vi "WPI_Robot6DriveMotors.vi"(8 "error in (no error)":errorcluster, 9 "RightSpeed":dbl, 10 "LeftSpeed":dbl, 11 "RobotDriveDevRef":T1={"DevStatus"={"status"=FALSE, "code"=0, "source"=""}, "Motors[]"=[], "Square Inputs"=FALSE, "Max Output"=1.0, "Isochronous"=FALSE}) -> (0 "error out":errorcluster, 2 "Motor Values":dbl[](array[numeric]), 3 "RobotDriveDevRef":T1={"DevStatus"={"status"=FALSE, "code"=0, "source"=""}, "Motors[]"=[], "Square Inputs"=FALSE, "Max Output"=1.0, "Isochronous"=FALSE})   [LabVIEW 2013]
doc: "Determines the motor configuration and sends the speed values to the appropriate motors.\n\nThis software is licensed. Open the labview\\readme\\WPI Robotics Library Open Source License.txt file for more information."
uses:
  <vilib>/Rock Robotics/WPI/RobotDrive/WPI_RobotDriveDevRef.ctl
  <vilib>/Rock Robotics/WPI/MotorControl/WPI_MotorControlDeviceRef.ctl
  <vilib>/Rock Robotics/SystemInterfaces/Typedef/FPGA_TypedefDigitalModule.ctl
  <vilib>/Rock Robotics/SystemInterfaces/DIO/FPGA_DIOPWMChannel.ctl
  <vilib>/Rock Robotics/WPI/PWM/WPI_PWMDeadband.ctl
  <vilib>/Rock Robotics/WPI/CAN/Jaguar/SubVIs/WPI_CANJaguar_ControlMode.ctl
  <vilib>/Rock Robotics/WPI/PWM/WPI_PWMTransform_ConPane.ctl
  WPI_RobotDriveMotorSelectorEnum.ctl
  <vilib>/Rock Robotics/WPI/RobotDrive/WPI_RobotDriveSafetyCheck.vi
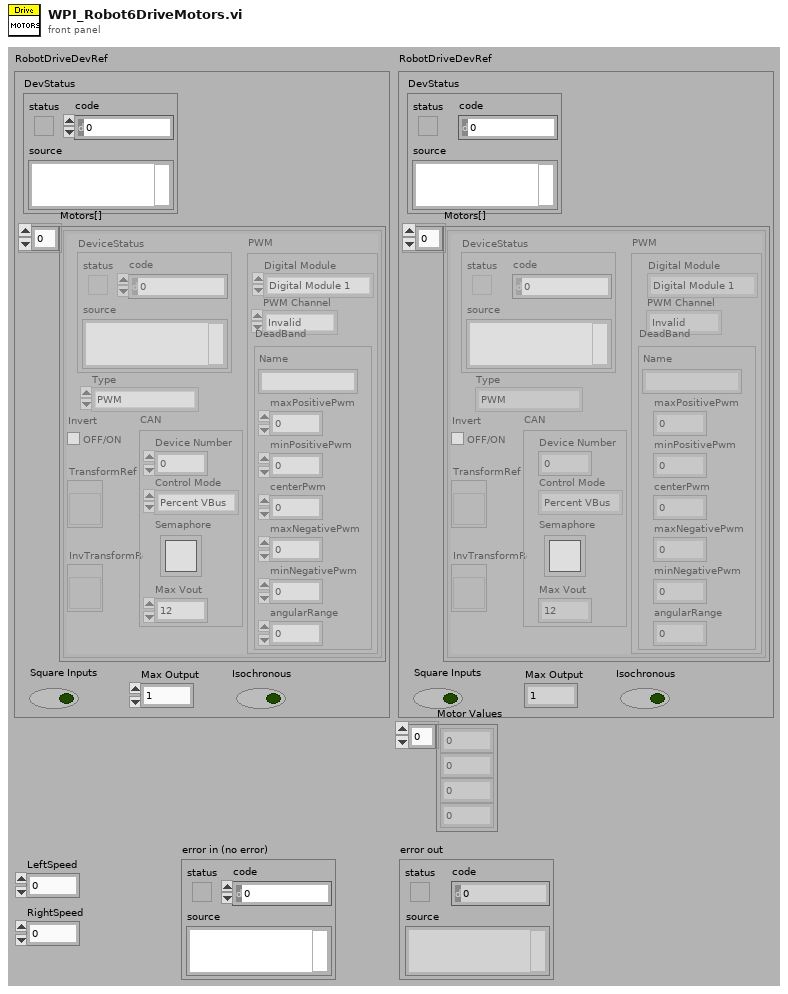
[diagram p1: front panel]
types:
  T1 = typedef "WPI_RobotDriveDevRef.ctl" = cluster{"DevStatus":errorcluster, "Motors[]":T2[], "Square Inputs":bool, "Max Output":dbl, "Isochronous":bool}
  T2 = typedef "WPI_MotorControlDeviceRef.ctl" = cluster{"DeviceStatus":errorcluster, "Type":enum16{"PWM", "CAN"}, "PWM":cluster{"Digital Module":T3, "PWM Channel":T4, "DeadBand":T5}, "CAN":cluster{"Device Number":u8, "Control Mode":T6, "Semaphore":T7, "Max Vout":dbl}, "Invert":bool, "TransformRef":T8, "InvTransformRef":T8}
  T3 = typedef "FPGA_TypedefDigitalModule.ctl" = enum16{"Digital Module 1", "Digital Module 2"}
  T4 = typedef "FPGA_DIOPWMChannel.ctl" = enum8{"PWM 1", "PWM 2", "PWM 3", "PWM 4", "PWM 5", "PWM 6", "PWM 7", "PWM 8", "PWM 9", "PWM 10", "Invalid"}
  T5 = typedef "WPI_PWMDeadband.ctl" = cluster{"Name":string, "maxPositivePwm":i32, "minPositivePwm":i32, "centerPwm":i32, "maxNegativePwm":i32, "minNegativePwm":i32, "angularRange":u16}
  T6 = typedef "WPI_CANJaguar_ControlMode.ctl" = enum8{"Percent VBus", "Current", "Speed", "Position", "Voltage"}
  T7 = typedef "Semaphore RefNum" = refnum<k1>
  T8 = typedef "WPI_PWMTransform_ConPane.ctl" = refnum<vi>
  T9 = typedef "WPI_RobotDriveMotorSelectorEnum.ctl" = enum16{"Rear Left Motor", "Rear Right Motor", "Front Left Motor", "Front Right Motor", "Mid Left Motor", "Mid Right Motor", ""}
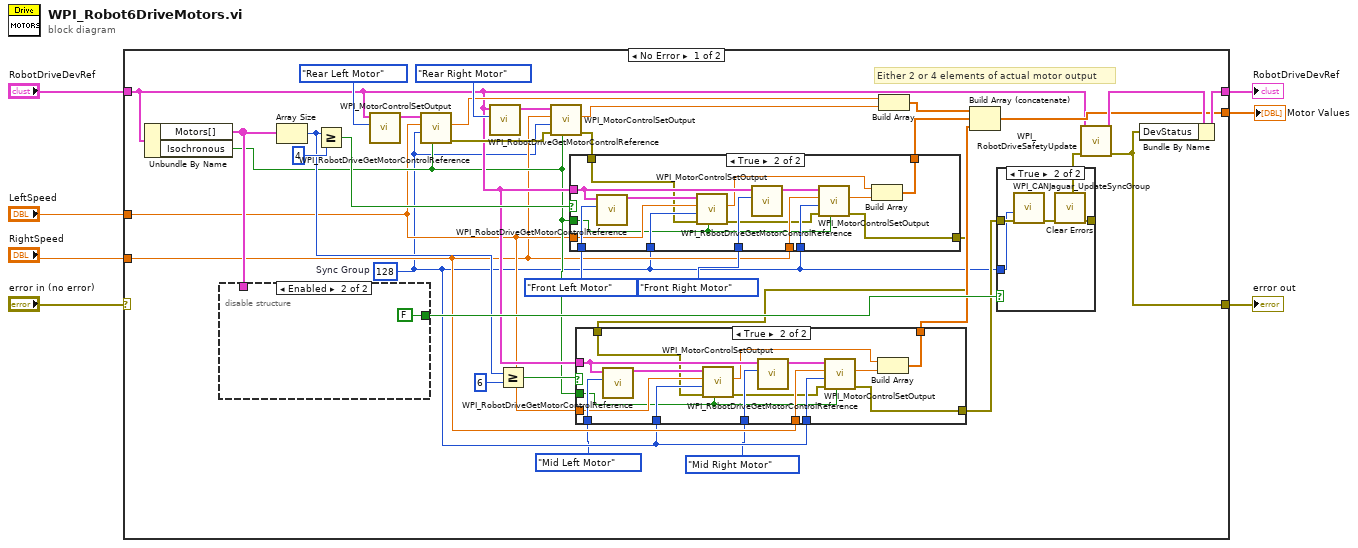
[diagram p0: block diagram]
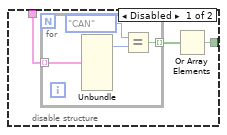
[diagram p2: hidden frame]
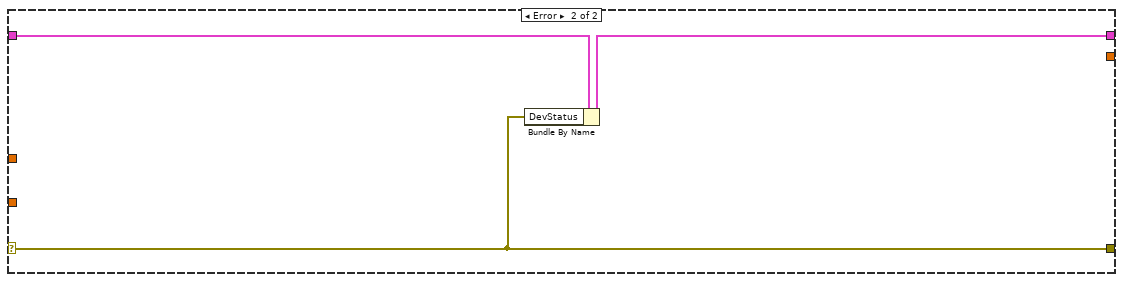
[diagram p6: hidden frame]
diagram:
  n1 = case shown="No Error" "error in (no error)" {
    selector: "error in (no error)" -> [_ w90]
    tunnel: "RobotDriveDevRef" -> [w18 w91]
    tunnel: [w32 w89] -> w6
    tunnel: "LeftSpeed" -> [w13 _]
    tunnel: "RightSpeed" -> [w12 _]
    tunnel: [w33 w90] -> w2
    tunnel: [w21 _] -> w1
    frame No Error {
      w11 = u8 128  # Sync Group
      # "Either 2 or 4 elements of actual motor output"
      n2 = Unbundle By Name(w18) -> ("Motors[]"=w30:T2[], "Isochronous"=w14:bool)
      n3 = disable-structure shown="Enabled" {
        disable-tunnel: w30 -> [w44 _]
        disable-tunnel: [w42 FALSE] -> w29
        frame Disabled {
          n4 = for {
            tunnel: w44 -> [w48] mode=indexing
            tunnel: [w45] -> w43 mode=indexing
            n5 = Unbundle(w48) -> ("Type"=w47:enum16{"PWM", "CAN"})  [unwired: 6 out]
            n6 = Equal?(x=enum16{"PWM", "CAN"}."CAN" ("Type"), y=w47) -> (x = y?=w45:bool)
          }
          n7 = Or Array Elements(Boolean array=w43) -> (logical OR=w42:bool)
        }
        frame Enabled {
        }
      }
      n8 = Array Size(array=w30) -> (size(s)=w19:i32)
      n9 = Greater Or Equal?(x=w19, y=4) -> (x >= y?=w31:bool)
      n10 = call <vilib>:"WPI_RobotDriveGetMotorControlReference.vi"("MotorIndex"=WPI_RobotDriveMotorSelectorEnum."Rear Left Motor", "RobotDriveDevRef"=w18) -> ("MotorControlDeviceRef"=w39:T2)  [unwired: 9 out]
      n11 = call <vilib>:"WPI_MotorControlSetOutput.vi"("Isochronous"=w14, "Sync Group"=w11, "Output"=w13, "MotorControlDevRef"=w39) -> ("error out"=w28:errorcluster, "Motor Output"=w25:dbl)  [unwired: 1 in, 5 out]
      n12 = call <vilib>:"WPI_RobotDriveGetMotorControlReference.vi"("MotorIndex"=WPI_RobotDriveMotorSelectorEnum."Rear Right Motor", "RobotDriveDevRef"=w18) -> ("MotorControlDeviceRef"=w40:T2)  [unwired: 9 out]
      n13 = Greater Or Equal?(x=w19, y=6) -> (x >= y?=w20:bool)
      n14 = call <vilib>:"WPI_MotorControlSetOutput.vi"("Isochronous"=w14, "error in (no error)"=w28, "Sync Group"=w11, "Output"=w12, "MotorControlDevRef"=w40) -> ("error out"=w27:errorcluster, "Motor Output"=w24:dbl)  [unwired: 5 out]
      n15 = case shown="True" w31 {
        tunnel: WPI_RobotDriveMotorSelectorEnum."Front Left Motor" ("MotorIndex") -> [_ w88]
        tunnel: WPI_RobotDriveMotorSelectorEnum."Front Right Motor" ("MotorIndex") -> [_ w87]
        tunnel: w18 -> [_ w86]
        tunnel: w11 -> [_ w85]
        tunnel: w12 -> [_ w84]
        tunnel: w13 -> [_ w83]
        tunnel: [w72 w78] -> w16
        tunnel: w11 -> [_ w80]
        tunnel: w14 -> [_ w79]
        tunnel: w27 -> [w72 w76]
        tunnel: [_ w73] -> w23
        frame False {
        }
        frame True {
          n16 = call <vilib>:"WPI_RobotDriveGetMotorControlReference.vi"("MotorIndex"=w88, "RobotDriveDevRef"=w86) -> ("MotorControlDeviceRef"=w81:T2)  [unwired: 9 out]
          n17 = call <vilib>:"WPI_MotorControlSetOutput.vi"("Isochronous"=w79, "error in (no error)"=w76, "Sync Group"=w80, "Output"=w83, "MotorControlDevRef"=w81) -> ("error out"=w77:errorcluster, "Motor Output"=w74:dbl)  [unwired: 5 out]
          n18 = call <vilib>:"WPI_RobotDriveGetMotorControlReference.vi"("MotorIndex"=w87, "RobotDriveDevRef"=w86) -> ("MotorControlDeviceRef"=w82:T2)  [unwired: 9 out]
          n19 = call <vilib>:"WPI_MotorControlSetOutput.vi"("Isochronous"=w79, "error in (no error)"=w77, "Sync Group"=w85, "Output"=w84, "MotorControlDevRef"=w82) -> ("error out"=w78:errorcluster, "Motor Output"=w75:dbl)  [unwired: 5 out]
          n20 = Build Array(w74, w75) -> (w73:dbl[])
        }
      }
      n21 = case shown="True" w20 {
        tunnel: WPI_RobotDriveMotorSelectorEnum."Mid Left Motor" ("MotorIndex") -> [_ w66]
        tunnel: WPI_RobotDriveMotorSelectorEnum."Mid Right Motor" ("MotorIndex") -> [_ w65]
        tunnel: w18 -> [_ w64]
        tunnel: w11 -> [_ w63]
        tunnel: w12 -> [_ w62]
        tunnel: w13 -> [_ w61]
        tunnel: [w50 w56] -> w15
        tunnel: w11 -> [_ w58]
        tunnel: w14 -> [_ w57]
        tunnel: w16 -> [w50 w54]
        tunnel: [_ w51] -> w17
        frame False {
        }
        frame True {
          n22 = call <vilib>:"WPI_RobotDriveGetMotorControlReference.vi"("MotorIndex"=w66, "RobotDriveDevRef"=w64) -> ("MotorControlDeviceRef"=w59:T2)  [unwired: 9 out]
          n23 = call <vilib>:"WPI_MotorControlSetOutput.vi"("Isochronous"=w57, "error in (no error)"=w54, "Sync Group"=w58, "Output"=w61, "MotorControlDevRef"=w59) -> ("error out"=w55:errorcluster, "Motor Output"=w52:dbl)  [unwired: 5 out]
          n24 = call <vilib>:"WPI_RobotDriveGetMotorControlReference.vi"("MotorIndex"=w65, "RobotDriveDevRef"=w64) -> ("MotorControlDeviceRef"=w60:T2)  [unwired: 9 out]
          n25 = call <vilib>:"WPI_MotorControlSetOutput.vi"("Isochronous"=w57, "error in (no error)"=w55, "Sync Group"=w63, "Output"=w62, "MotorControlDevRef"=w60) -> ("error out"=w56:errorcluster, "Motor Output"=w53:dbl)  [unwired: 5 out]
          n26 = Build Array(w52, w53) -> (w51:dbl[])
        }
      }
      n27 = Build Array(w25, w24) -> (w22:dbl[])
      n28 = Build Array (concatenate)(w22, w23, w17) -> (w21:dbl[])
      n29 = case shown="True" w29 {
        tunnel: w15 -> [w67 w70]
        tunnel: w11 -> [_ w69]
        tunnel: [w67 w68] -> w26
        frame False {
        }
        frame True {
          n30 = call <vilib>:"WPI_CANJaguar_UpdateSyncGroup.vi"("error in (no error)"=w70, "Sync Group"=w69) -> ("error out"=w71:errorcluster)  [unwired: 9 out]
          n31 = call <vilib>:"Clear Errors.vi"("error in (no error)"=w71) -> ("error out"=w68:errorcluster)  [unwired: 6 out]
        }
      }
      n32 = call <vilib>:"WPI_RobotDriveSafetyUpdate.vi"("error in (no error)"=w26, "RobotDriveDevRef"=w18) -> ("error out"=w33:errorcluster, "RobotDriveDevRef"=w34:T1)  [unwired: 8 out]
      n33 = Bundle By Name(cluster=w34, "DevStatus"=w33) -> (w32:T1)
    }
    frame Error {
      n34 = Bundle By Name(cluster=w91, "DevStatus"=w90) -> (w89:T1)
    }
  }
  "RobotDriveDevRef" <- w6
  "error out" <- w2
  "Motor Values" <- w1
